vi "Equal Value.vi"(0 "result":bool, 1 "Slot":i32, 3 "timeout ms (-1)":i32, 5 "X":string, 7 "Station":T1(ring), 9 "Y":string, 11 "error in (no error)":errorcluster, 12 "Unit":string, 13 "type":T2, 14 "StepName":string) -> (15 "error out":errorcluster)   [LabVIEW 2019, in "Unit Test Engine Tools.lvlib"]
uses:
  Unit Test Engine Tools.lvlib
  <vilib>/Utility/Data Type/Type Definitions/Data Type.ctl
  e59ab1b6-8b9e-43b0-9d77-13d228640eb2.vi
  LVUT Global 1.vi
  <resource>/objmgr/ni.dex.rc
  <vilib>/Utility/Data Type/NI_Data Type.lvlib
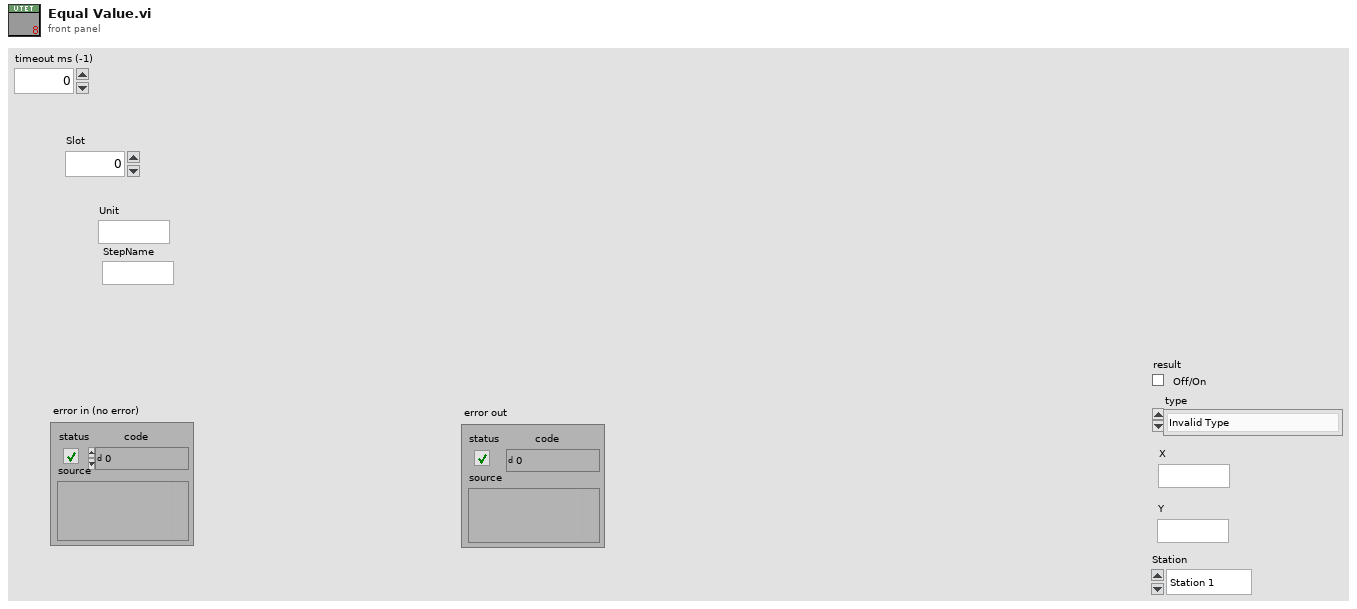
[diagram p1: front panel]
types:
  T1 = enum16{"Station 1", "Station 2", "Station 3", "Station 4"}
  T2 = typedef "NI_Data Type.lvlib/Data Type.ctl" = enum8{"Invalid Type", "Void", "I8", "I16", "I32", "I64", "U8", "U16", "U32", "U64", "Single Float", "Double Float", "Extended Float", "Single Complex", "Double Complex", "Extended Complex", "Enum U8", "Enum U16", "Enum U32", "Enum U64", "Single Float With Unit", "Double Float With Unit", "Extended Float With Unit", "Single Complex with Unit", "Double Complex with Unit", "Extended Complex with Unit", "Boolean", "String", "Path", "Picture", "Tag", "Array", "Cluster", "Variant", "LV Variant", "Waveform", "Timestamp", "Digital Waveform", "Digital Data", "ExpressData", "Refnum", "External Data", "VI", "Poly VI", "LabVIEW Class Instance", "Fixed Point", "Set Collection", "Map Collection"}
  T3 = cluster{"Slot":i32, string, "X":string, cluster{"Y":string, "Y":string}, "RingText.Text":string, "StepName":string, "Y":string, "Unit":string}
  T4 = cluster{"Slot":i32, "Result":string, "Value":string, "Limit":cluster{"High":string, "Low":string}, "Type":string, "StepName":string, "Normal":string, "Unit":string}
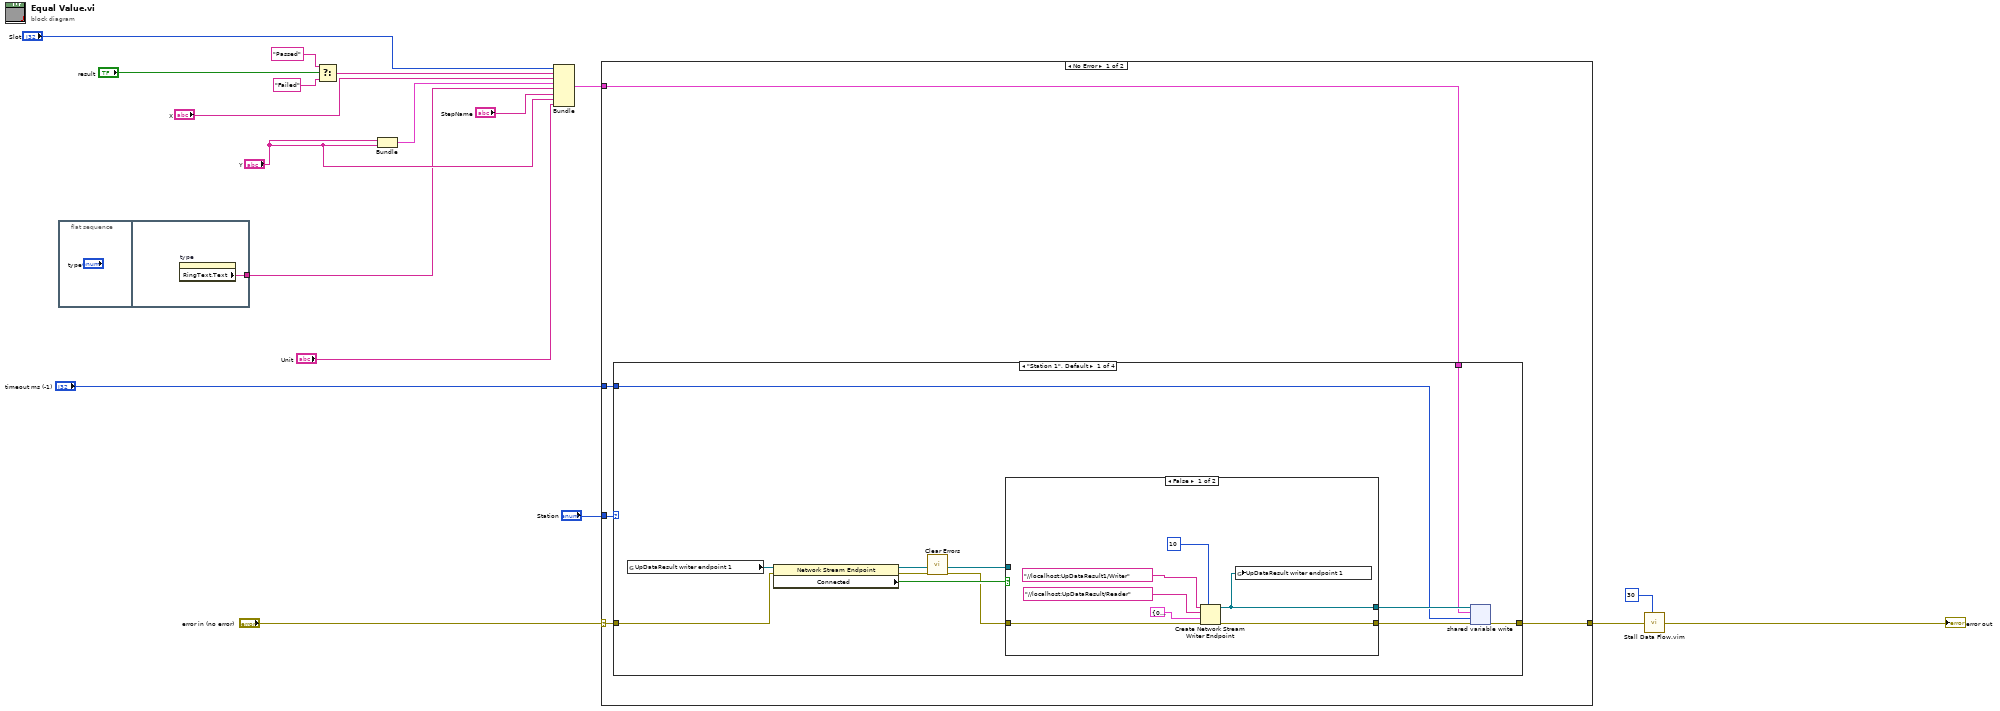
[diagram p0: block diagram]
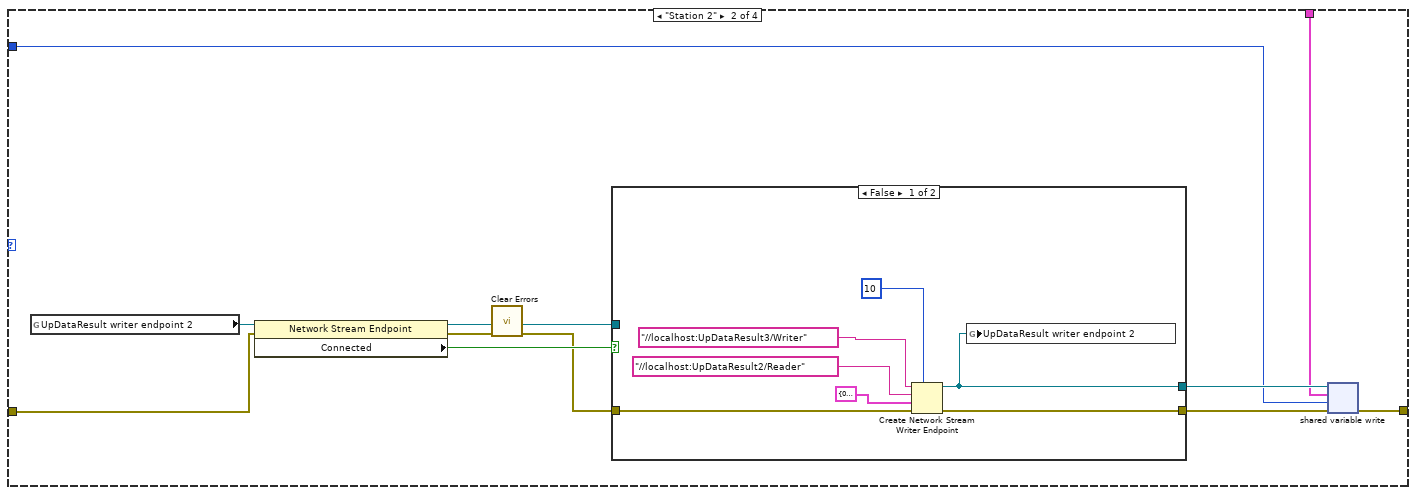
[diagram p3: hidden frame]
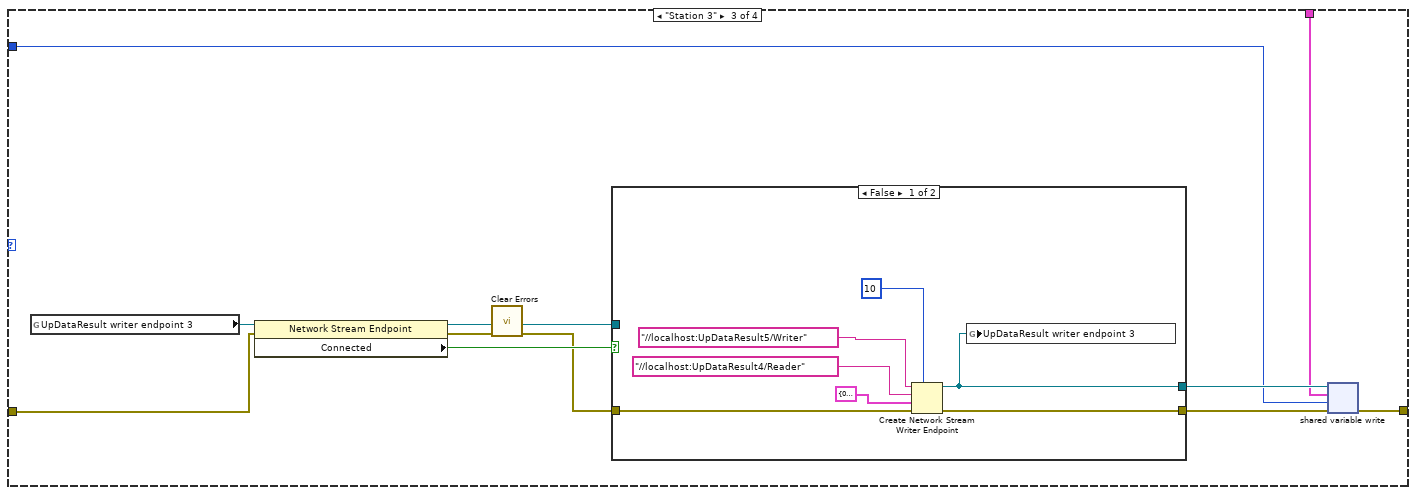
[diagram p5: hidden frame]
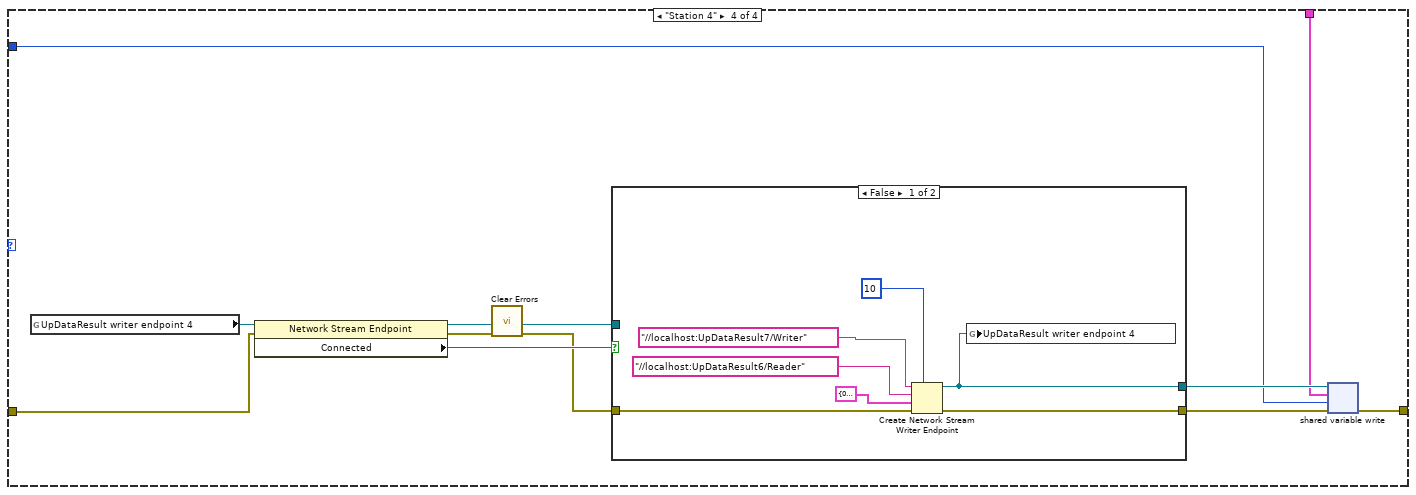
[diagram p7: hidden frame]
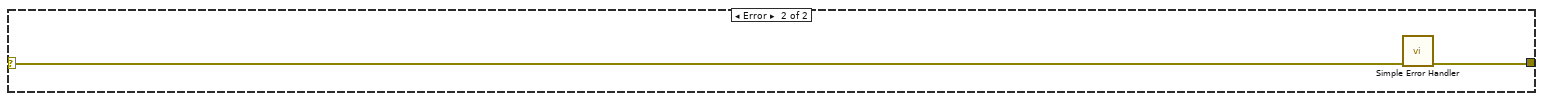
[diagram p9: hidden frame]
diagram:
  n1 = flat-sequence {
    tunnel: [w19] -> w2
    frame #0 {
    }
    frame #1 {
      n2 = property on="type" class="Enum (strict)"() -> ("RingText.Text"=w19:string)  [unwired: 2 in, 2 out]
    }
  }
  n3 = Select(t="Passed", s="result", f="Failed") -> (s? t:f=w15:string)
  n4 = Bundle("Y"="Y", "Y"="Y") -> (w14:cluster{"Y":string, "Y":string})  [unwired: 1 in]
  n5 = Bundle("Slot"="Slot", w15, "X"="X", w14, "RingText.Text"=w2, "StepName"="StepName", "Y"="Y", "Unit"="Unit") -> (w10:T3)  [unwired: 1 in]
  n6 = case shown="No Error" "error in (no error)" {
    selector: "error in (no error)" -> [w21 w106]
    tunnel: "timeout ms (-1)" -> [w24 _]
    tunnel: w10 -> [w23 _]
    tunnel: [w22 w105] -> w8
    tunnel: "Station" -> [w20 _]
    frame No Error {
      n7 = case shown="\"Station 1\", Default" w20 {
        tunnel: w24 -> [w33 w53 w73 w93]
        tunnel: w23 -> [w32 w52 w72 w92]
        tunnel: [w27 w47 w67 w87] -> w22
        tunnel: w21 -> [w26 w46 w66 w86]
        frame "Station 1", Default {
          n8 = global read "LVUT Global 1.vi" "UpDataResult writer endpoint 1"() -> (w31:refnum<k21>)
          n9 = property class="Network Stream Endpoint"(reference=w31, error in=w26) -> (reference out=w28:refnum<k21>, error out=w30:errorcluster, "Connected"=w29:bool)
          n10 = call <vilib>:"Clear Errors.vi"("error in (no error)"=w30) -> ("error out"=w25:errorcluster)  [unwired: 5 in, 1 out]
          n11 = case shown="False" w29 {
            tunnel: [w36 w44] -> w35
            tunnel: [w41 w43] -> w34
            tunnel: w25 -> [w37 w43]
            tunnel: w28 -> [_ w44]
            frame False {
              n12 = Create Network Stream Writer Endpoint(7:10 ("writer buffer size"), 8:w37, 9:T4 {"Slot"=0, "Result"="", "Value"="", "Limit"={"High"="", "Low"=""}, "Type"="", "StepName"="", "Normal"="", "Unit"=""}, 10:"//localhost:UpDataResult/Reader" ("reader name"), 11:"//localhost:UpDataResult1/Writer" ("reader name")) -> (0:w41:errorcluster, 3:w36:refnum<k21>)  [unwired: 2 in]
              n13 = global write "LVUT Global 1.vi" "UpDataResult writer endpoint 1"(w36) -> ()
            }
            frame True {
            }
          }
          n14 = shared-variable-write(w35, w34, w32, w33) -> (w27:errorcluster)  [unwired: 2 out]
        }
        frame "Station 2" {
          n15 = global read "LVUT Global 1.vi" "UpDataResult writer endpoint 2"() -> (w51:refnum<k21>)
          n16 = property class="Network Stream Endpoint"(reference=w51, error in=w46) -> (reference out=w48:refnum<k21>, error out=w50:errorcluster, "Connected"=w49:bool)
          n17 = call <vilib>:"Clear Errors.vi"("error in (no error)"=w50) -> ("error out"=w45:errorcluster)  [unwired: 5 in, 1 out]
          n18 = case shown="False" w49 {
            tunnel: [w56 w64] -> w55
            tunnel: [w61 w63] -> w54
            tunnel: w45 -> [w57 w63]
            tunnel: w48 -> [_ w64]
            frame False {
              n19 = Create Network Stream Writer Endpoint(7:10 ("writer buffer size"), 8:w57, 9:T4 {"Slot"=0, "Result"="", "Value"="", "Limit"={"High"="", "Low"=""}, "Type"="", "StepName"="", "Normal"="", "Unit"=""}, 10:"//localhost:UpDataResult2/Reader" ("reader name"), 11:"//localhost:UpDataResult3/Writer" ("reader name")) -> (0:w61:errorcluster, 3:w56:refnum<k21>)  [unwired: 2 in]
              n20 = global write "LVUT Global 1.vi" "UpDataResult writer endpoint 2"(w56) -> ()
            }
            frame True {
            }
          }
          n21 = shared-variable-write(w55, w54, w52, w53) -> (w47:errorcluster)  [unwired: 2 out]
        }
        frame "Station 3" {
          n22 = global read "LVUT Global 1.vi" "UpDataResult writer endpoint 3"() -> (w71:refnum<k21>)
          n23 = property class="Network Stream Endpoint"(reference=w71, error in=w66) -> (reference out=w68:refnum<k21>, error out=w70:errorcluster, "Connected"=w69:bool)
          n24 = call <vilib>:"Clear Errors.vi"("error in (no error)"=w70) -> ("error out"=w65:errorcluster)  [unwired: 5 in, 1 out]
          n25 = case shown="False" w69 {
            tunnel: [w76 w84] -> w75
            tunnel: [w81 w83] -> w74
            tunnel: w65 -> [w77 w83]
            tunnel: w68 -> [_ w84]
            frame False {
              n26 = Create Network Stream Writer Endpoint(7:10 ("writer buffer size"), 8:w77, 9:T4 {"Slot"=0, "Result"="", "Value"="", "Limit"={"High"="", "Low"=""}, "Type"="", "StepName"="", "Normal"="", "Unit"=""}, 10:"//localhost:UpDataResult4/Reader" ("reader name"), 11:"//localhost:UpDataResult5/Writer" ("reader name")) -> (0:w81:errorcluster, 3:w76:refnum<k21>)  [unwired: 2 in]
              n27 = global write "LVUT Global 1.vi" "UpDataResult writer endpoint 3"(w76) -> ()
            }
            frame True {
            }
          }
          n28 = shared-variable-write(w75, w74, w72, w73) -> (w67:errorcluster)  [unwired: 2 out]
        }
        frame "Station 4" {
          n29 = global read "LVUT Global 1.vi" "UpDataResult writer endpoint 4"() -> (w91:refnum<k21>)
          n30 = property class="Network Stream Endpoint"(reference=w91, error in=w86) -> (reference out=w88:refnum<k21>, error out=w90:errorcluster, "Connected"=w89:bool)
          n31 = call <vilib>:"Clear Errors.vi"("error in (no error)"=w90) -> ("error out"=w85:errorcluster)  [unwired: 5 in, 1 out]
          n32 = case shown="False" w89 {
            tunnel: [w96 w104] -> w95
            tunnel: [w101 w103] -> w94
            tunnel: w85 -> [w97 w103]
            tunnel: w88 -> [_ w104]
            frame False {
              n33 = Create Network Stream Writer Endpoint(7:10 ("writer buffer size"), 8:w97, 9:T4 {"Slot"=0, "Result"="", "Value"="", "Limit"={"High"="", "Low"=""}, "Type"="", "StepName"="", "Normal"="", "Unit"=""}, 10:"//localhost:UpDataResult6/Reader" ("reader name"), 11:"//localhost:UpDataResult7/Writer" ("reader name")) -> (0:w101:errorcluster, 3:w96:refnum<k21>)  [unwired: 2 in]
              n34 = global write "LVUT Global 1.vi" "UpDataResult writer endpoint 4"(w96) -> ()
            }
            frame True {
            }
          }
          n35 = shared-variable-write(w95, w94, w92, w93) -> (w87:errorcluster)  [unwired: 2 out]
        }
      }
    }
    frame Error {
      n36 = call <vilib>:"Simple Error Handler.vi"("error in (no error)"=w106) -> ("error out"=w105:errorcluster)  [unwired: 4 in, 4 out]
    }
  }
  n37 = call "Stall Data Flow.vim"("value in"=w8, "milliseconds to wait"=u32 30) -> ("value out"=→"error out":errorcluster)  [unwired: 1 out]
